vi "GetVIXML.vi"(11 "VI Path":string) -> (2 "Output":string, 3 "Error Code":i32)   [LabVIEW 2026]
doc: "This vi adds two number for valid inputs."
uses:
  <vilib>/Utility/Symbolic Paths/NI_SymbolicPaths.lvlib
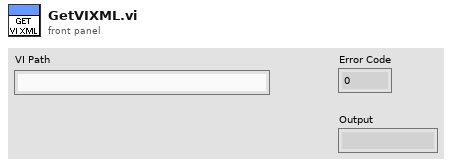
[diagram p1: front panel]
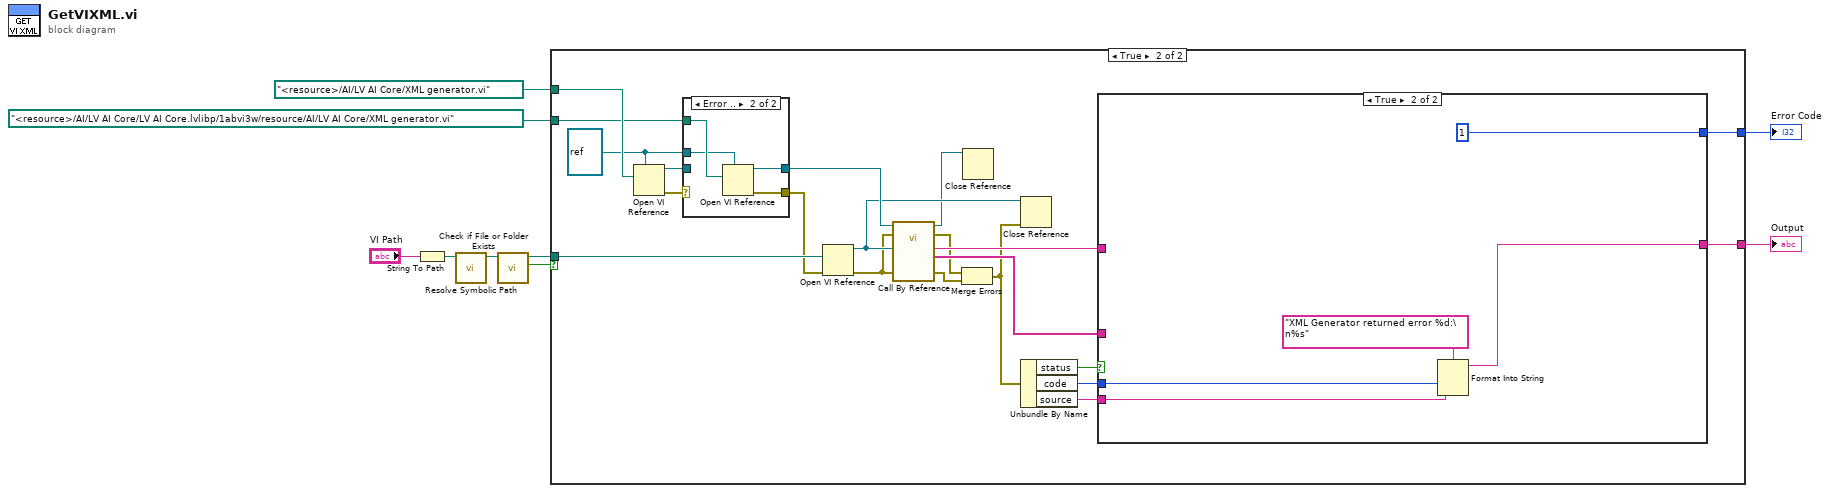
[diagram p0: block diagram]
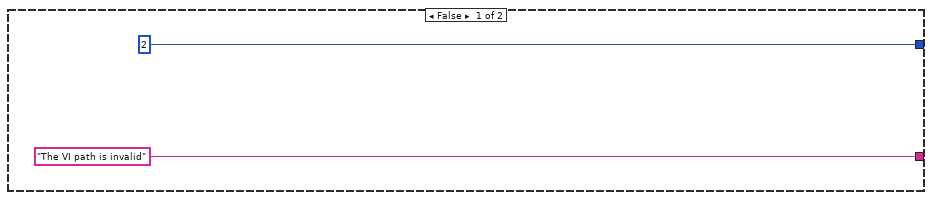
[diagram p2: hidden frame]
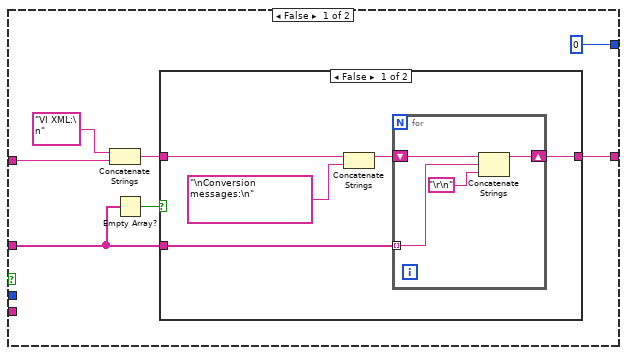
[diagram p4: hidden frame]
diagram:
  n1 = String To Path(string="VI Path") -> (path=w2:path)
  n2 = call <vilib>:"Resolve Symbolic Path.vi"("path"=w2) -> ("resolved path"=w1:path)  [unwired: 8 in, 2 out]
  n3 = call <vilib>:"Check if File or Folder Exists.vi"("path"=w1) -> ("file or folder exists?"=w7:bool, "dup path"=w6:path)  [unwired: 8 in, 1 out]
  n4 = case shown="True" w7 {
    tunnel: [2 w27] -> w8
    tunnel: ["The VI path is invalid" w30] -> w9
    tunnel: w6 -> [_ w32]
    tunnel: path "<resource>/AI/LV AI Core/XML generator.vi" ("vi path") -> [_ w26]
    tunnel: path "<resource>/AI/LV AI Core/LV AI Core.lvlibp/1abvi3w/resource/AI/LV AI Core/XML generator.vi" ("vi path") -> [_ w24]
    frame False {
    }
    frame True {
      w22 = refnum<vi> refnum ("type specifier VI Refnum (for type only)")
      n5 = Open VI Reference(type specifier VI Refnum (for type only)=w22, vi path=w26) -> (vi reference=w23:refnum<vi>, error out=w25:errorcluster)  [unwired: 4 in]
      n6 = case shown="Error .." w25 {
        selector: w25 -> [w34 _]
        tunnel: [w34 w38] -> w21
        tunnel: [w33 w37] -> w20
        tunnel: w24 -> [_ w36]
        tunnel: w23 -> [w33 _]
        tunnel: w22 -> [_ w35]
        frame No Error {
        }
        frame Error {
          n7 = Open VI Reference(type specifier VI Refnum (for type only)=w35, vi path=w36) -> (vi reference=w37:refnum<vi>, error out=w38:errorcluster)  [unwired: 4 in]
        }
      }
      n8 = Open VI Reference(vi path=w32, error in (no error)=w21) -> (vi reference=w19:refnum<vi>, error out=w12:errorcluster)  [unwired: 4 in]
      n9 = call-by-ref "?"(reference=w20, error in=w12, 8:"error in (no error)"=w12, "vi"=w19) -> (reference out=w13:refnum<vi>, error out=w15:errorcluster, 0:"error out"=w16:errorcluster, "conversion messages"=w17:string[], "XML (UTF-8 encoded)"=w18:string)  [unwired: 6 in, 1 out]
      n10 = Merge Errors(w15, w16) -> (w14:errorcluster)
      n11 = Close Reference(reference=w13) -> ()  [unwired: 1 in, 1 out]
      n12 = Close Reference(reference=w19, error in (no error)=w14) -> ()  [unwired: 1 out]
      n13 = Unbundle By Name(w14) -> ("status"=w31:bool, "code"=w29:i32, "source"=w28:string)
      n14 = case shown="True" w31 {
        tunnel: w18 -> [w44 _]
        tunnel: w17 -> [w42 _]
        tunnel: [w40 w57] -> w30
        tunnel: w29 -> [_ w60]
        tunnel: w28 -> [_ w59]
        tunnel: [0 1] -> w27
        frame False {
          n15 = Concatenate Strings("VI XML:\n", w44) -> (w43:string)
          n16 = Empty Array?(array=w42) -> (empty?=w41:bool)
          n17 = case shown="False" w41 {
            tunnel: w43 -> [w49 w55]
            tunnel: w42 -> [w50 _]
            tunnel: [w46 w55] -> w40
            frame False {
              n18 = Concatenate Strings(w49, "\nConversion messages:\n") -> (w47:string)
              n19 = for {
                tunnel: w50 -> [w53] mode=indexing
                shift-right: [w51] -> w46
                shift-left: w47 -> [w54]
                n20 = Concatenate Strings(w54, w53, "\r\n") -> (w51:string)
              }
            }
            frame True {
            }
          }
        }
        frame True {
          n21 = Format Into String(format string="XML Generator returned error %d:\n%s", w60, w59) -> (resulting string=w57:string)  [unwired: 2 in, 1 out]
        }
      }
    }
  }
  "Error Code" <- w8
  "Output" <- w9
